vi "Convert_InstrumentReferenceArray_2_ChannelReferenceArray.vi"(2 "error in (no error)":errorcluster, 3 "DCPowerInformationClusterArray_Input":T1[](array[typedef])) -> (0 "error out":errorcluster, 1 "DCPowerInformationArrayOutput":T2(array[cluster]))   [LabVIEW 2019]
uses:
  Controls/DCPowerBlock_byInstrument_Control.ctl
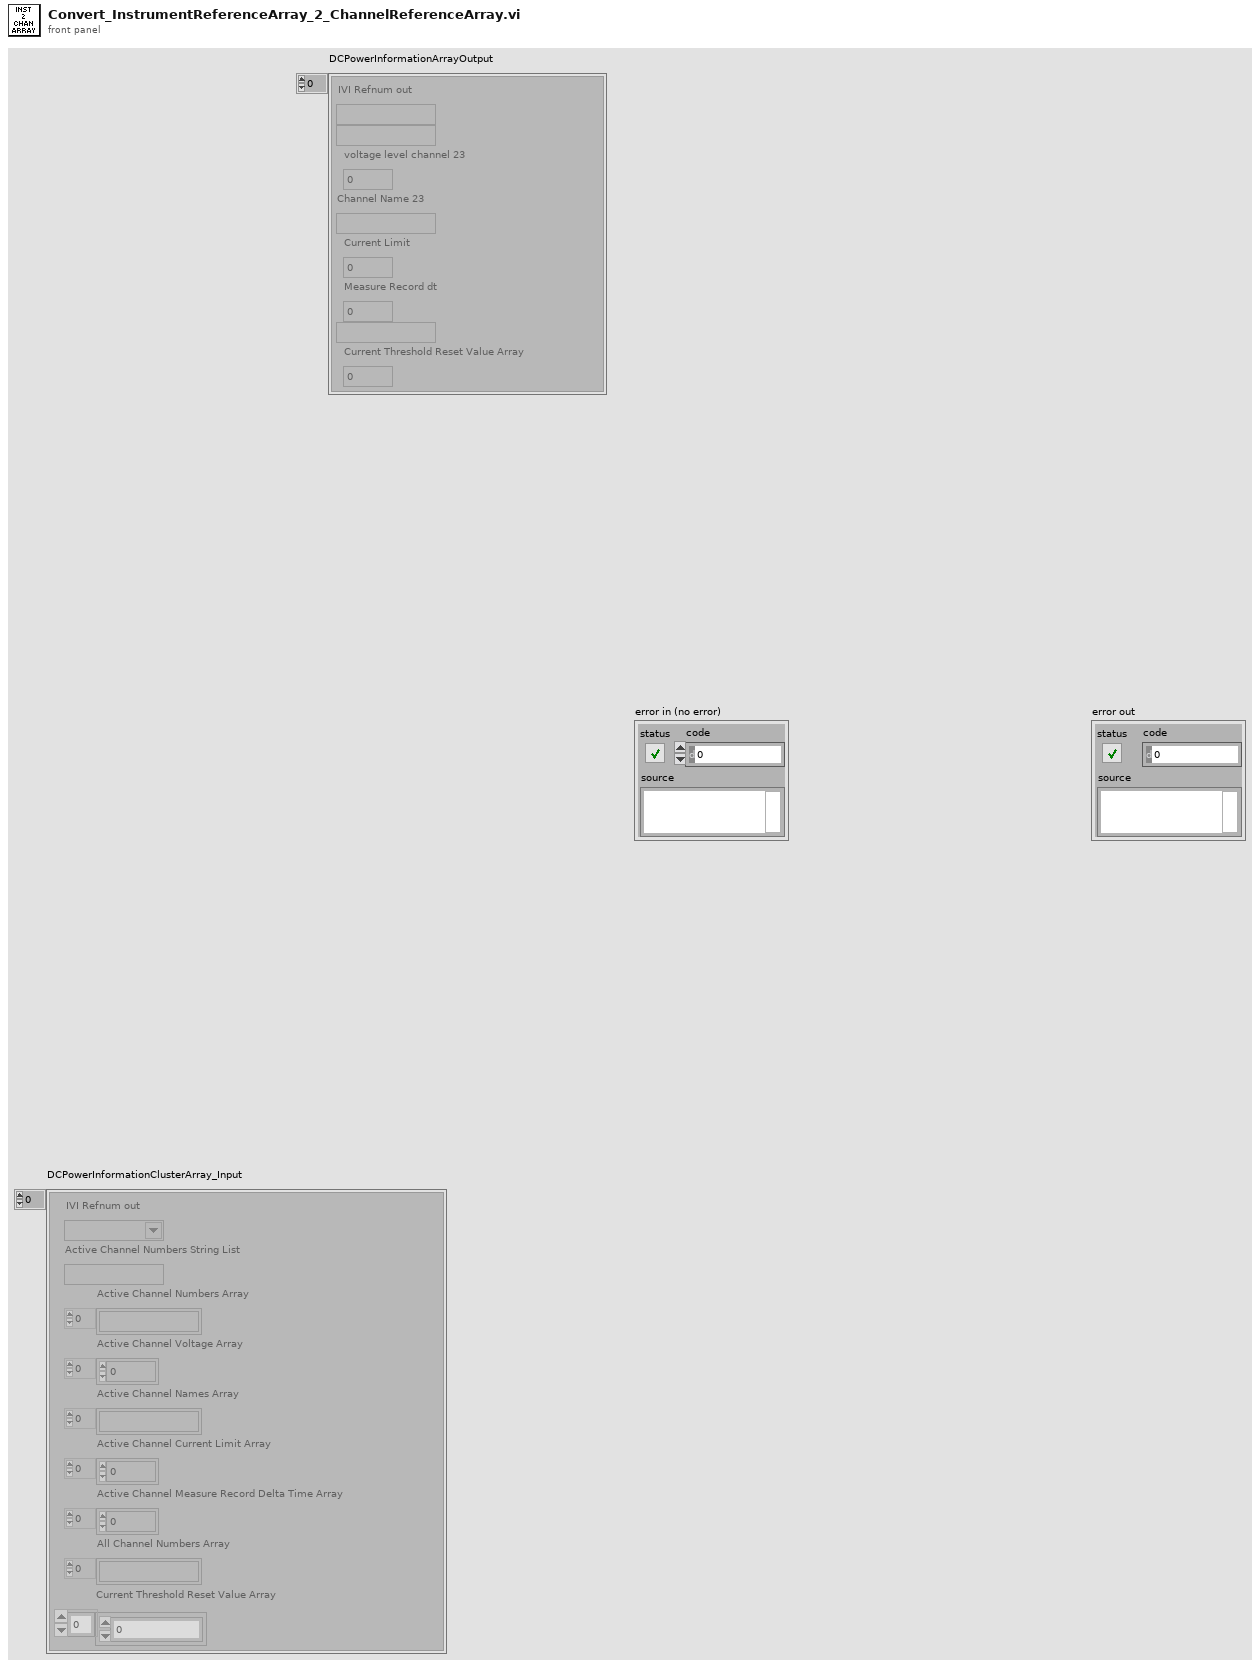
[diagram p1: front panel]
types:
  T1 = typedef "DCPowerBlock_byInstrument_Control.ctl" = cluster{"IVI Refnum out":refnum<k15>, "Active Channel Numbers String List":string, "Active Channel Numbers Array":string[], "Active Channel Voltage Array":dbl[], "Active Channel Names Array":string[], "Active Channel Current Limit Array":dbl[], "Active Channel Measure Record Delta Time Array":dbl[], "All Channel Numbers Array":string[], "Current Threshold Reset Value Array":dbl[]}
  T2 = cluster{"IVI Refnum out":refnum<k15>, string, "voltage level channel 23":dbl, "Channel Name 23":string, "Current Limit":dbl, "Measure Record dt":dbl, string, "Current Threshold Reset Value Array":dbl}[]
  T3 = cluster{"IVI Refnum out":refnum<k15>, string, "voltage level channel 23":dbl, "Channel Name 23":string, "Current Limit":dbl, "Measure Record dt":dbl, void}
  T4 = cluster{"IVI Refnum out":refnum<k15>, string, "voltage level channel 23":dbl, "Channel Name 23":string, "Current Limit":dbl, "Measure Record dt":dbl, string, "Current Threshold Reset Value Array":dbl}
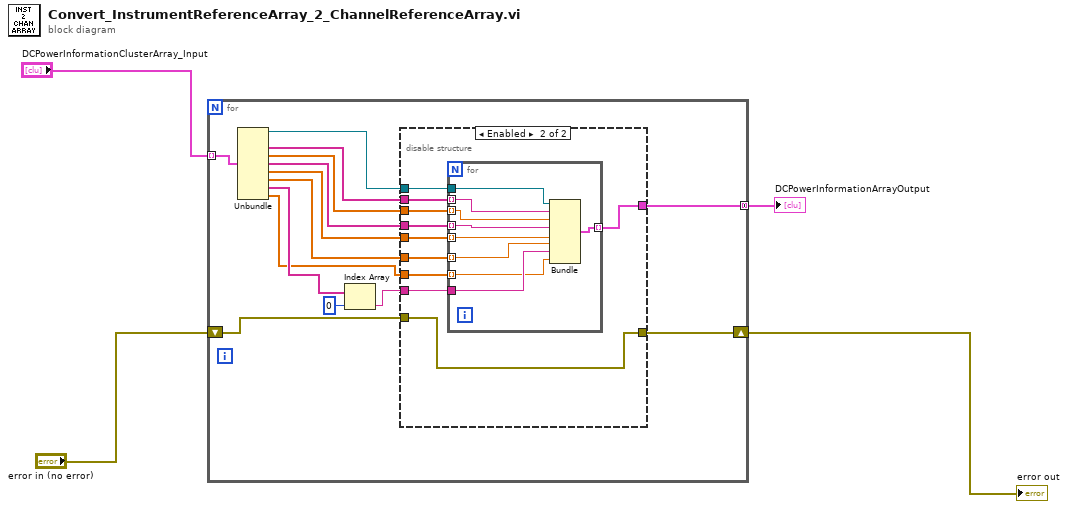
[diagram p0: block diagram]
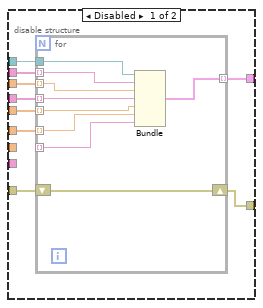
[diagram p2: hidden frame]
diagram:
  n1 = for {
    tunnel: "DCPowerInformationClusterArray_Input" -> [w18] mode=indexing
    tunnel: [w15] -> w2 mode=concatenating
    shift-right: [w14] -> w4
    shift-left: "error in (no error)" -> [w13]
    n2 = Unbundle(w18) -> ("IVI Refnum out"=w17:refnum<k15>, "Active Channel Numbers Array"=w16:string[], "Active Channel Voltage Array"=w12:dbl[], "Active Channel Names Array"=w11:string[], "Active Channel Current Limit Array"=w10:dbl[], "Active Channel Measure Record Delta Time Array"=w9:dbl[], "All Channel Numbers Array"=w8:string[], "Current Threshold Reset Value Array"=w5:dbl[])  [unwired: 1 out]
    n3 = Index Array(array=w8, index=0) -> (element=w6:string)
    n4 = disable-structure shown="Enabled" {
      disable-tunnel: w17 -> [w27 w41]
      disable-tunnel: w16 -> [w26 w42]
      disable-tunnel: [w25 w40] -> w15
      disable-tunnel: [w24 w39] -> w14
      disable-tunnel: w13 -> [w23 w39]
      disable-tunnel: w12 -> [w22 w43]
      disable-tunnel: w11 -> [w21 w44]
      disable-tunnel: w10 -> [w20 w45]
      disable-tunnel: w9 -> [w19 w46]
      disable-tunnel: w6 -> [_ w38]
      disable-tunnel: w5 -> [_ w37]
      frame Disabled {
        n5 = for {
          tunnel: w27 -> [w36]
          tunnel: w26 -> [w33] mode=indexing
          tunnel: [w35] -> w25 mode=indexing
          shift-right: [w34] -> w24
          shift-left: w23 -> [w34]
          tunnel: w22 -> [w32] mode=indexing
          tunnel: w21 -> [w31] mode=indexing
          tunnel: w20 -> [w30] mode=indexing
          tunnel: w19 -> [w29] mode=indexing
          tunnel: _ -> [w28] mode=indexing
          n6 = Bundle("IVI Refnum out"=w36, w33, "voltage level channel 23"=w32, "Channel Name 23"=w31, "Current Limit"=w30, "Measure Record dt"=w29, w28) -> (w35:T3)  [unwired: 1 in]
        }
      }
      frame Enabled {
        n7 = for {
          tunnel: w46 -> [w55] mode=indexing
          tunnel: w45 -> [w54] mode=indexing
          tunnel: w44 -> [w53] mode=indexing
          tunnel: w43 -> [w52] mode=indexing
          tunnel: w42 -> [w51] mode=indexing
          tunnel: w41 -> [w50]
          tunnel: [w49] -> w40 mode=indexing
          tunnel: w38 -> [w48]
          tunnel: w37 -> [w47] mode=indexing
          n8 = Bundle("IVI Refnum out"=w50, w51, "voltage level channel 23"=w52, "Channel Name 23"=w53, "Current Limit"=w54, "Measure Record dt"=w55, w48, "Current Threshold Reset Value Array"=w47) -> (w49:T4)  [unwired: 1 in]
        }
      }
    }
  }
  "error out" <- w4
  "DCPowerInformationArrayOutput" <- w2
